vi "Charger_Is Ready.vi"(6 "Stop Refnum":refnum<vi>, 7 "Status Refnum":T1, 8 "error in":errorcluster) -> (0 "error out":errorcluster, 2 "ready":bool)   [LabVIEW 2020]
doc: "If the input error status is FALSE (no error) and the STOP control refnum value is TRUE, then this function puts the message \"Terminated by user at x:xx AM/PM.\" with the current time in the error message cluster and sets the error status to TRUE. \n\nIf the input error status is TRUE (error) the existing error cluster is unchanged."
uses:
  Charger_Status Refnum.ctl
  Drivers/Charger Test Set/Charger_Input Control.ctl
panel:
  out "stop":bool
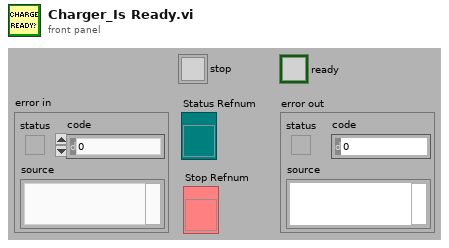
[diagram p1: front panel]
types:
  T1 = typedef "Charger_Status Refnum.ctl" = refnum<vi>
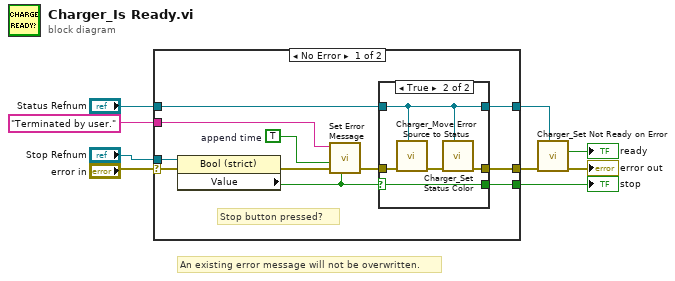
[diagram p0: block diagram]
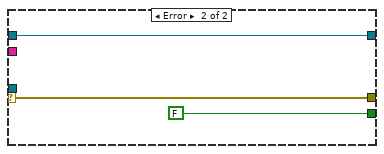
[diagram p3: hidden frame]
diagram:
  # "An existing error message will not be overwritten."
  n1 = case shown="No Error" "error in" {
    selector: "error in" -> [w15 w30]
    tunnel: "Stop Refnum" -> [w19 _]
    tunnel: [w13 w30] -> w3
    tunnel: "Terminated by user." ("Message") -> [w18 _]
    tunnel: "Status Refnum" -> [w10 w28]
    tunnel: [w11 FALSE] -> w5
    tunnel: [w10 w28] -> w2
    frame No Error {
      w16 = TRUE  # append time
      # "Stop button pressed?"
      n2 = property class="Bool (strict)"(reference=w19, error in=w15) -> (error out=w17:errorcluster, "Value"=w12:bool)  [unwired: 1 out]
      n3 = call "Set Error Message.vi"("enable (T)"=w12, "error in"=w17, "append time (F)"=w16, "message"=w18) -> ("error out"=w14:errorcluster)  [unwired: 4 in]
      n4 = case shown="True" w12 {
        selector: w12 -> [w22 w26]
        tunnel: w14 -> [w21 w25]
        tunnel: [w21 w27] -> w13
        tunnel: [w22 w26] -> w11
        tunnel: [w20 w23] -> _
        tunnel: w10 -> [w20 w23]
        frame False {
        }
        frame True {
          n5 = call "Charger_Move Error Source to Status.vi"("error in"=w25, "Status Refnum"=w23) -> ("error out"=w24:errorcluster)  [unwired: 8 in]
          n6 = call "Charger_Set Status Color.vi"("error in"=w24, "Status Refnum"=w23) -> ("error out"=w27:errorcluster)  [unwired: 8 in]
        }
      }
    }
    frame Error {
    }
  }
  "stop" <- w5
  n7 = call "Charger_Set Not Ready on Error.vi"("Status Refnum"=w2, "error in"=w3) -> ("error out"=→"error out":errorcluster, "ready status"=→"ready":bool)  [unwired: 7 in]
